vi "Omit_Rows_Containing_new.vi"(2 "Data Array In":string[][](array[string]), 3 "Non-Blank Rows":i32[](array[numeric]), 4 "Template Info":string[][](array[string])) -> (0 "Row numbers":i32[](array[numeric]), 1 "Data Array Out":string[][](array[string]))   [LabVIEW 2010]
panel:
  out "No of Rows Removed":i32
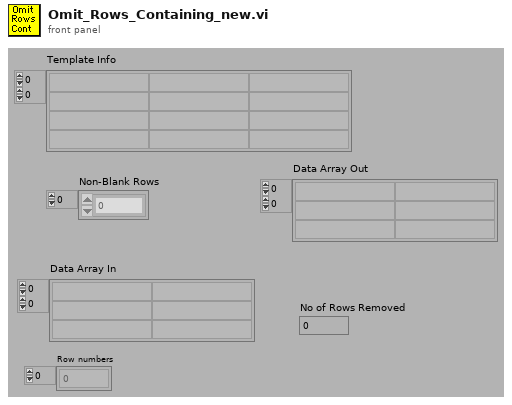
[diagram p1: front panel]
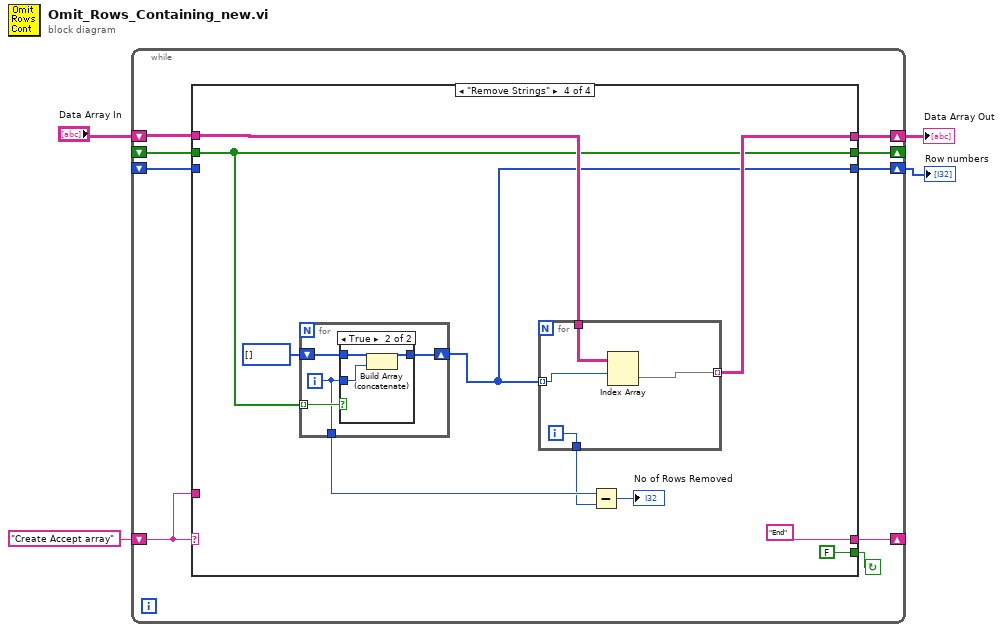
[diagram p0: block diagram]
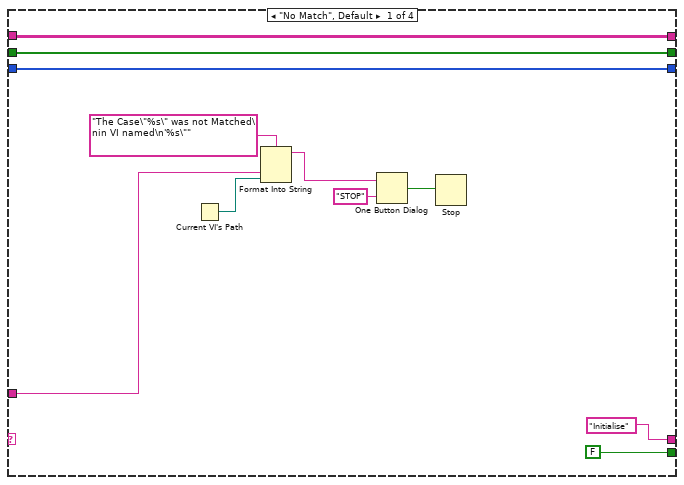
[diagram p2: hidden frame]
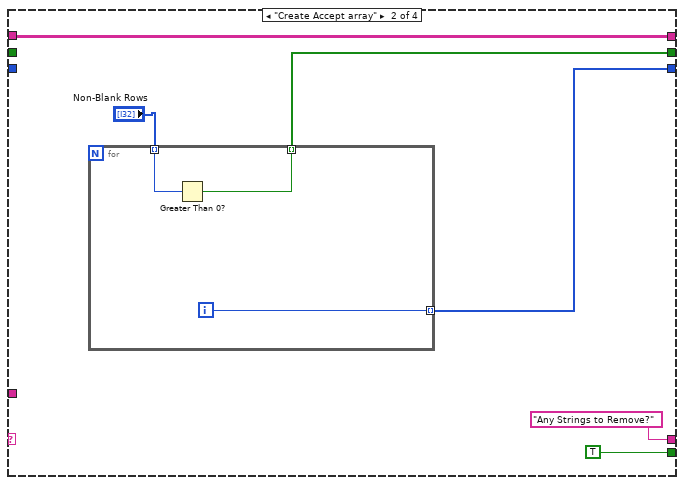
[diagram p3: hidden frame]
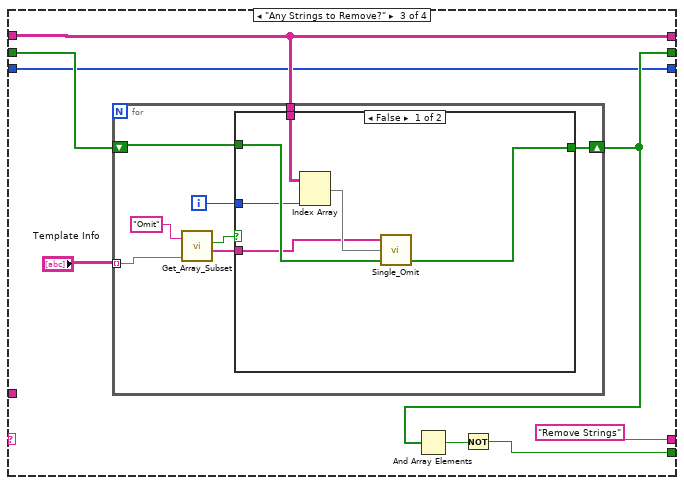
[diagram p4: hidden frame]
diagram:
  n1 = while {
    shift-left: _ -> [w7]
    shift-right: [w8] -> _
    shift-left: "Data Array In" -> [w10]
    shift-right: [w9] -> w2
    shift-left: "Create Accept array" -> [w11]
    shift-right: [w12] -> _
    shift-right: [w6] -> w1
    shift-left: _ -> [w5]
    stop <- w13 continue-if-true
    n2 = case shown="\"Remove Strings\"" w11 {
      tunnel: [FALSE TRUE w35 FALSE] -> w13
      tunnel: ["Initialise" "Any Strings to Remove?" "Remove Strings" "End"] -> w12
      tunnel: w11 -> [w19 _ _ _]
      tunnel: w10 -> [w16 w26 w38 w64]
      tunnel: [w16 w26 w38 w63] -> w9
      tunnel: [w15 w28 w37 w62] -> w8
      tunnel: w7 -> [w15 _ w39 w62]
      tunnel: [w14 w27 w34 w57] -> w6
      tunnel: w5 -> [w14 _ w34 _]
      frame "No Match", Default {
        n3 = Current VI's Path() -> (path=w18:path)
        n4 = Format Into String(format string="The Case\"%s\" was not Matched\nin VI named\n'%s\"" ("Format String"), w19, w18) -> (resulting string=w22:string)  [unwired: 2 in, 1 out]
        n5 = One Button Dialog(message=w22, button name ("OK")="STOP") -> (true=w20:bool)
        n6 = Stop(stop? (T)=w20) -> ()
      }
      frame "Create Accept array" {
        n7 = for {
          tunnel: [w31] -> w28 mode=indexing
          tunnel: [w33] -> w27 mode=indexing
          tunnel: "Non-Blank Rows" -> [w32] mode=indexing
          i -> [w33]
          n8 = Greater Than 0?(x=w32) -> (x > 0?=w31:bool)
        }
      }
      frame "Any Strings to Remove?" {
        n9 = for {
          tunnel: "Template Info" -> [w48] mode=indexing
          shift-right: [w45] -> w37
          shift-left: w39 -> [w46]
          tunnel: w38 -> [w42]
          i -> [w43]
          n10 = call "Get_Array_Subset.vi"("String Array In"=w48, "Subset Name"="Omit") -> ("Array Subset Out"=w44:string[], "Empty Subset?"=w47:bool)  [unwired: 3 out]
          n11 = case shown="False" w47 {
            tunnel: w46 -> [w55 w56]
            tunnel: [w54 w56] -> w45
            tunnel: w44 -> [w50 _]
            tunnel: w43 -> [w53 _]
            tunnel: w42 -> [w52 _]
            frame False {
              n12 = Index Array(array=w52, index (col)=w53) -> (element=w51:string[])  [unwired: 1 in]
              n13 = call "Single_Omit.vi"("Accept In"=w55, "Data Values"=w51, "Omit Strings"=w50) -> ("Accept Out"=w54:bool[])  [unwired: 2 out]
            }
            frame True {
            }
          }
        }
        n14 = And Array Elements(Boolean array=w37) -> (logical AND=w36:bool)
        n15 = Not(x=w36) -> (.not. x?=w35:bool)
      }
      frame "Remove Strings" {
        n16 = for {
          shift-right: [w73] -> w57
          shift-left: i32[] [] -> [w72]
          tunnel: w62 -> [w74] mode=indexing
          tunnel: [w71] -> w60
          i -> [w71]
          n17 = case shown="True" w74 {
            tunnel: w71 -> [_ w77]
            tunnel: [w75 w76] -> w73
            tunnel: w72 -> [w75 w78]
            frame False {
            }
            frame True {
              n18 = Build Array (concatenate)(w78, w77) -> (w76:i32[])
            }
          }
        }
        n19 = for {
          tunnel: w57 -> [w68] mode=indexing
          tunnel: w64 -> [w70]
          tunnel: [w69] -> w63 mode=indexing
          tunnel: [w67] -> w59
          i -> [w67]
          n20 = Index Array(array=w70, index (row)=w68) -> (element=w69:string[])  [unwired: 1 in]
        }
        n21 = Subtract(x=w60, y=w59) -> (x-y=→"No of Rows Removed":i32)
      }
    }
  }
  "Data Array Out" <- w2
  "Row numbers" <- w1
